vi "calculate starts.vi"(0 "Tomo in":refnum<class "Tomo.lvclass">, 11 "error in (no error)":errorcluster) -> (3 "x loop number":i32, 4 "Tomo out":refnum<class "Tomo.lvclass">, 6 "x_start":dbl[unit], 8 "y_start":dbl[unit], 10 "step size":dbl[unit], 14 "y loop number":i32, 15 "error out":errorcluster)   [LabVIEW 2012, in "Tomo.lvclass"]
uses:
  Tomo.lvclass
  Tomo.lvclass/Tomo.ctl
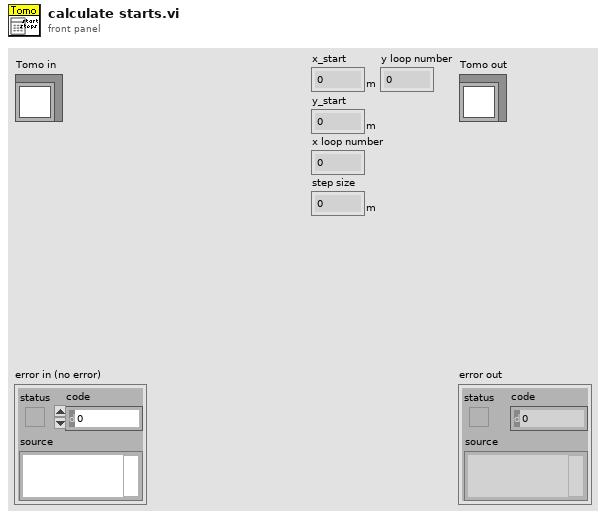
[diagram p1: front panel]
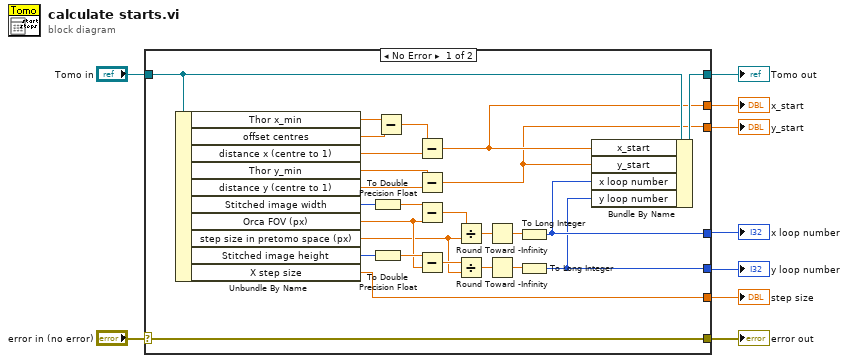
[diagram p0: block diagram]
diagram:
  n1 = case shown="No Error" "error in (no error)" {
    selector: "error in (no error)" -> [w35 w37]
    tunnel: [w35 w37] -> w8
    tunnel: [w29 w36] -> w6
    tunnel: "Tomo in" -> [w30 w36]
    tunnel: [w26 _] -> w5
    tunnel: [w24 _] -> w4
    tunnel: [w13 _] -> w3
    tunnel: [w12 _] -> w2
    tunnel: [w10 _] -> w1
    frame No Error {
      n2 = Unbundle By Name(w30) -> ("Thor x_min"=w33:dbl[unit], "offset centres"=w34:dbl[unit], "distance x (centre to 1)"=w31:dbl[unit], "Thor y_min"=w28:dbl[unit], "distance y (centre to 1)"=w27:dbl[unit], "Stitched image width"=w25:i32, "Orca FOV (px)"=w17:dbl, "step size in pretomo space (px)"=w11:dbl, "Stitched image height"=w19:i32, "X step size"=w10:dbl[unit])
      n3 = To Double Precision Float(number=w25) -> (double precision float=w23:dbl)
      n4 = To Double Precision Float(number=w19) -> (double precision float=w18:dbl)
      n5 = Subtract(x=w33, y=w34) -> (x-y=w32:dbl[unit])
      n6 = Subtract(x=w32, y=w31) -> (x-y=w26:dbl[unit])
      n7 = Subtract(x=w28, y=w27) -> (x-y=w24:dbl[unit])
      n8 = Subtract(x=w23, y=w17) -> (x-y=w22:dbl)
      n9 = Subtract(x=w18, y=w17) -> (x-y=w14:dbl)
      n10 = Divide(x=w22, y=w11) -> (x/y=w21:dbl)
      n11 = Divide(x=w14, y=w11) -> (x/y=w15:dbl)
      n12 = Round Toward -Infinity(1:w21) -> (0:w20:dbl)
      n13 = Round Toward -Infinity(1:w15) -> (0:w16:dbl)
      n14 = To Long Integer(number=w20) -> (32bit integer=w13:i32)
      n15 = To Long Integer(number=w16) -> (32bit integer=w12:i32)
      n16 = Bundle By Name(cluster=w30, "x_start"=w26, "y_start"=w24, "x loop number"=w13, "y loop number"=w12) -> (w29:refnum<class "Tomo.lvclass">)
    }
    frame Error {
    }
  }
  "error out" <- w8
  "Tomo out" <- w6
  "x_start" <- w5
  "y_start" <- w4
  "x loop number" <- w3
  "y loop number" <- w2
  "step size" <- w1
